vi "Get settings chain.vi"(8 "error in (no error)":errorcluster, 11 "Test_ExampleClassA in":refnum<class "Test_ExampleClassA.lvclass">) -> (0 "error out":errorcluster, 1 "class name":string[](array[string]), 2 "settings":variant[](array[variant]), 3 "Test_ExampleClassA out":refnum<class "Test_ExampleClassA.lvclass">)   [LabVIEW 2012, in "Test_ExampleClassA.lvclass"]
doc: "Returns an array of variants containing the settings clusters of each class in the inheritance chain (lowest child class first), together with an array of all class names in the inheritance chain.\n\nFor classes without settings cluster, the settings chain contains empty variants."
uses:
  Test_ExampleClassA.lvclass
  MurmexTest/MurmexTest.lvclass
  Murmex/Murmex.lvclass
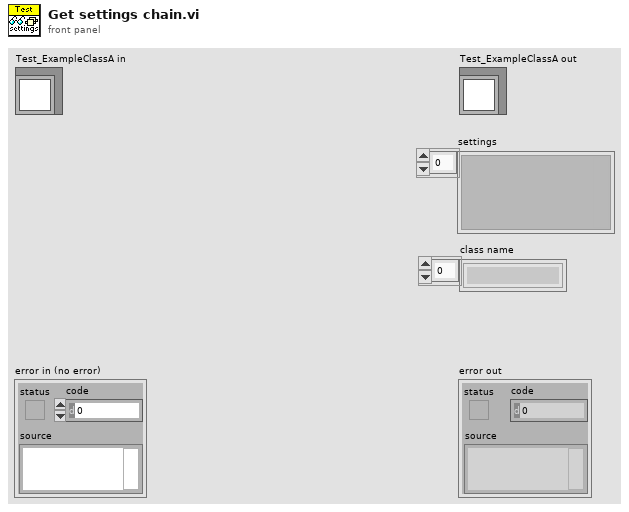
[diagram p1: front panel]
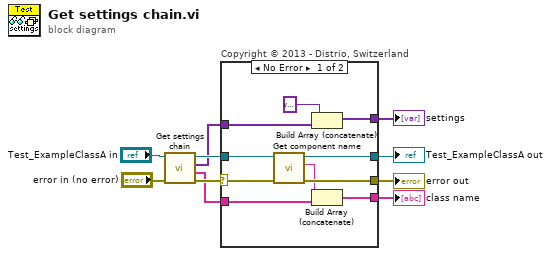
[diagram p0: block diagram]
diagram:
  n1 = call-parent "Get settings chain.vi"("error in (no error)"="error in (no error)", "MurmexTest in"="Test_ExampleClassA in") -> ("error out"=w8:errorcluster, "class name"=w5:string[], "settings"=w6:variant[], "MurmexTest out"=w7:refnum<class "Test_ExampleClassA.lvclass">)  [unwired: 6 in]
  n2 = case "Copyright © 2013 - Distrio, Switzerland" shown="No Error" w8 {
    selector: w8 -> [w18 w22]
    tunnel: [w20 w22] -> w1
    tunnel: [w16 _] -> w2
    tunnel: [w15 _] -> w4
    tunnel: [w19 w21] -> w3
    tunnel: w7 -> [w12 w21]
    tunnel: w6 -> [w13 _]
    tunnel: w5 -> [w14 _]
    frame No Error {
      n3 = call "Get component name.vi"("error in (no error)"=w18, "Murmex in"=w12) -> ("error out"=w20:errorcluster, "component name"=w17:string, "Murmex out"=w19:refnum<class "Test_ExampleClassA.lvclass">)  [unwired: 7 in]
      n4 = Build Array (concatenate)(variant ("Variant"), w13) -> (w15:variant[])
      n5 = Build Array (concatenate)(w17, w14) -> (w16:string[])
    }
    frame Error {
    }
  }
  "error out" <- w1
  "Test_ExampleClassA out" <- w3
  "settings" <- w4
  "class name" <- w2
